vi "Main_FPGA 4.vi"() -> ()   [LabVIEW 2015]
uses:
  <vilib>/LabVIEW Targets/FPGA/cRIO/shared/nicrio_ModuleControls/nicrio_cRIO-9232_ConfigModeRing.ctl
  <vilib>/rvi/Emulation/niFpgaGetClockAttributes.vi
  <vilib>/rvi/Emulation/niFpgaSctlEmulationGetInTimedLoop.vi
  <vilib>/rvi/Emulation/niFpgaEmulationReportErrorSimple.vi
  <vilib>/rvi/Emulation/niFpgaProcessEmulError.vi
  <vilib>/rvi/eio/common/nirviEmuTemplateMethod_errors.vi
  <vilib>/rvi/interface/RandomDataEmulation/niFpgaRandomDataHandleErrors.vi
  <vilib>/rvi/Emulation/niFpgaCriticalErrorInLSC.vi
  <vilib>/eio/EIONode/EIONode.xnode
  <vilib>/rvi/DataTransferAndStorage/Container/XNode/niFpgaContainer.xnode
  <vilib>/rvi/interface/RandomDataEmulation/nirviRandomDataFpgaReadWriteTemplate.vi
  <vilib>/addons/InsightCM/Devices/Shared/AcquireBOP/FPGA/subVIs/VibAPI/BOP_VibAPI_6.lvlib
panel:
  out "Loop delay (us)":u32
  out "Chassis Temperature":sgl
  in  "Custom Scale Intercept":sgl[](array[numeric])=[0.0, 0.0, 0.0, 0.0, 0.0, 0.0, 0.0, 0.0, 0.0, 0.0, 0.0, 0.0, 0.0, 0.0, 0.0, 0.0, 0.0, 0.0, 0.0, 0.0, 0.0, 0.0, 0.0, 0.0, 0.0, 0.0, 0.0, 0.0, 0.0, 0.0, 0.0, 0.0, 0.0, 0.0, 0.0, 0.0, 0.0, 0.0, 0.0, 0.0, 0.0, 0.0, 0.0, 0.0, 0.0, 0.0, 0.0, 0.0, 0.0, 0.0, 0.0, 0.0, 0.0, 0.0, 0.0, 0.0, 0.0, 0.0, 0.0, 0.0, 0.0, 0.0, 0.0, 0.0, 0.0, 0.0, 0.0, 0.0, 0.0, 0.0, 0.0, 0.0, 0.0, 0.0, 0.0, 0.0, 0.0, 0.0, 0.0, 0.0, 0.0, 0.0, 0.0, 0.0, 0.0, 0.0, 0.0, 0.0, 0.0, 0.0, 0.0, 0.0, 0.0, 0.0, 0.0, 0.0, 0.0, 0.0, 0.0, 0.0, 0.0, 0.0, 0.0, 0.0, 0.0, 0.0, 0.0, 0.0, 0.0, 0.0, 0.0, 0.0, 0.0, 0.0, 0.0, 0.0, 0.0, 0.0, 0.0, 0.0, 0.0, 0.0, 0.0, 0.0, 0.0, 0.0, 0.0, 0.0]
  out "FPGA Error":errorcluster
  out "Finished":bool
  in  "Stop":bool
  out "Module Underflow":bool
  out "DMA FIFO Full":bool
  out "Chan Count":bool
  out "Acq Loop Ticks":u32
  out "First Read":bool
  in  "Total Avail Channels":i32=4
  in  "Data Rate [S/s]":u32=1280
  in  "Custom Scale Slope":sgl[](array[numeric])=[0.0, 0.0, 0.0, 0.0, 0.0, 0.0, 0.0, 0.0, 0.0, 0.0, 0.0, 0.0, 0.0, 0.0, 0.0, 0.0, 0.0, 0.0, 0.0, 0.0, 0.0, 0.0, 0.0, 0.0, 0.0, 0.0, 0.0, 0.0, 0.0, 0.0, 0.0, 0.0, 0.0, 0.0, 0.0, 0.0, 0.0, 0.0, 0.0, 0.0, 0.0, 0.0, 0.0, 0.0, 0.0, 0.0, 0.0, 0.0, 0.0, 0.0, 0.0, 0.0, 0.0, 0.0, 0.0, 0.0, 0.0, 0.0, 0.0, 0.0, 0.0, 0.0, 0.0, 0.0, 0.0, 0.0, 0.0, 0.0, 0.0, 0.0, 0.0, 0.0, 0.0, 0.0, 0.0, 0.0, 0.0, 0.0, 0.0, 0.0, 0.0, 0.0, 0.0, 0.0, 0.0, 0.0, 0.0, 0.0, 0.0, 0.0, 0.0, 0.0, 0.0, 0.0, 0.0, 0.0, 0.0, 0.0, 0.0, 0.0, 0.0, 0.0, 0.0, 0.0, 0.0, 0.0, 0.0, 0.0, 0.0, 0.0, 0.0, 0.0, 0.0, 0.0, 0.0, 0.0, 0.0, 0.0, 0.0, 0.0, 0.0, 0.0, 0.0, 0.0, 0.0, 0.0, 0.0, 0.0]
  in  "Acquisition Type":enum16{"Finite Samples", "Continuous Samples"}(ring)
  in  "Samps per Chan [Finite]":i32=5120
  in  "Input Config Array":T1[](array[typedef])=[0, 0, 0, 0, 0, 0, 0, 0, 0, 0, 0, 0, 0, 0, 0, 0, 0, 0, 0, 0, 0, 1, 1, 1] items=["AC Coupled", "DC Coupled", "IEPE AC Coupled"]
  in  "Number of Modules":i16=1
  in  "Enable Chan Array":bool[](array[boolean])
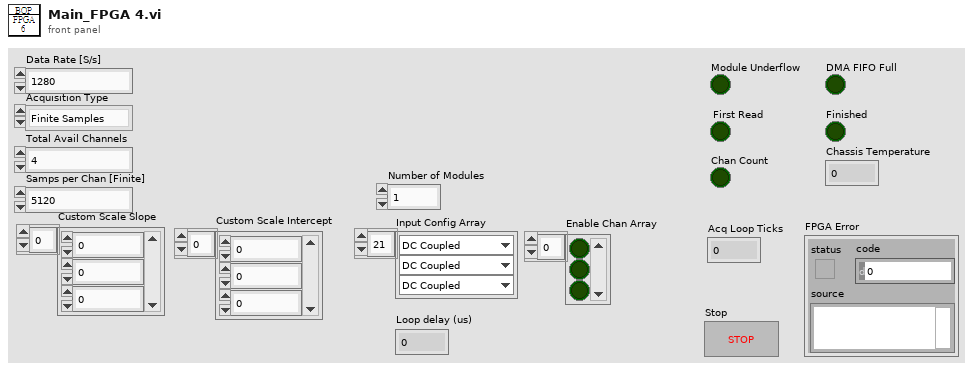
[diagram p1: front panel]
types:
  T1 = typedef "nicrio_cRIO-9232_ConfigModeRing.ctl" = u8
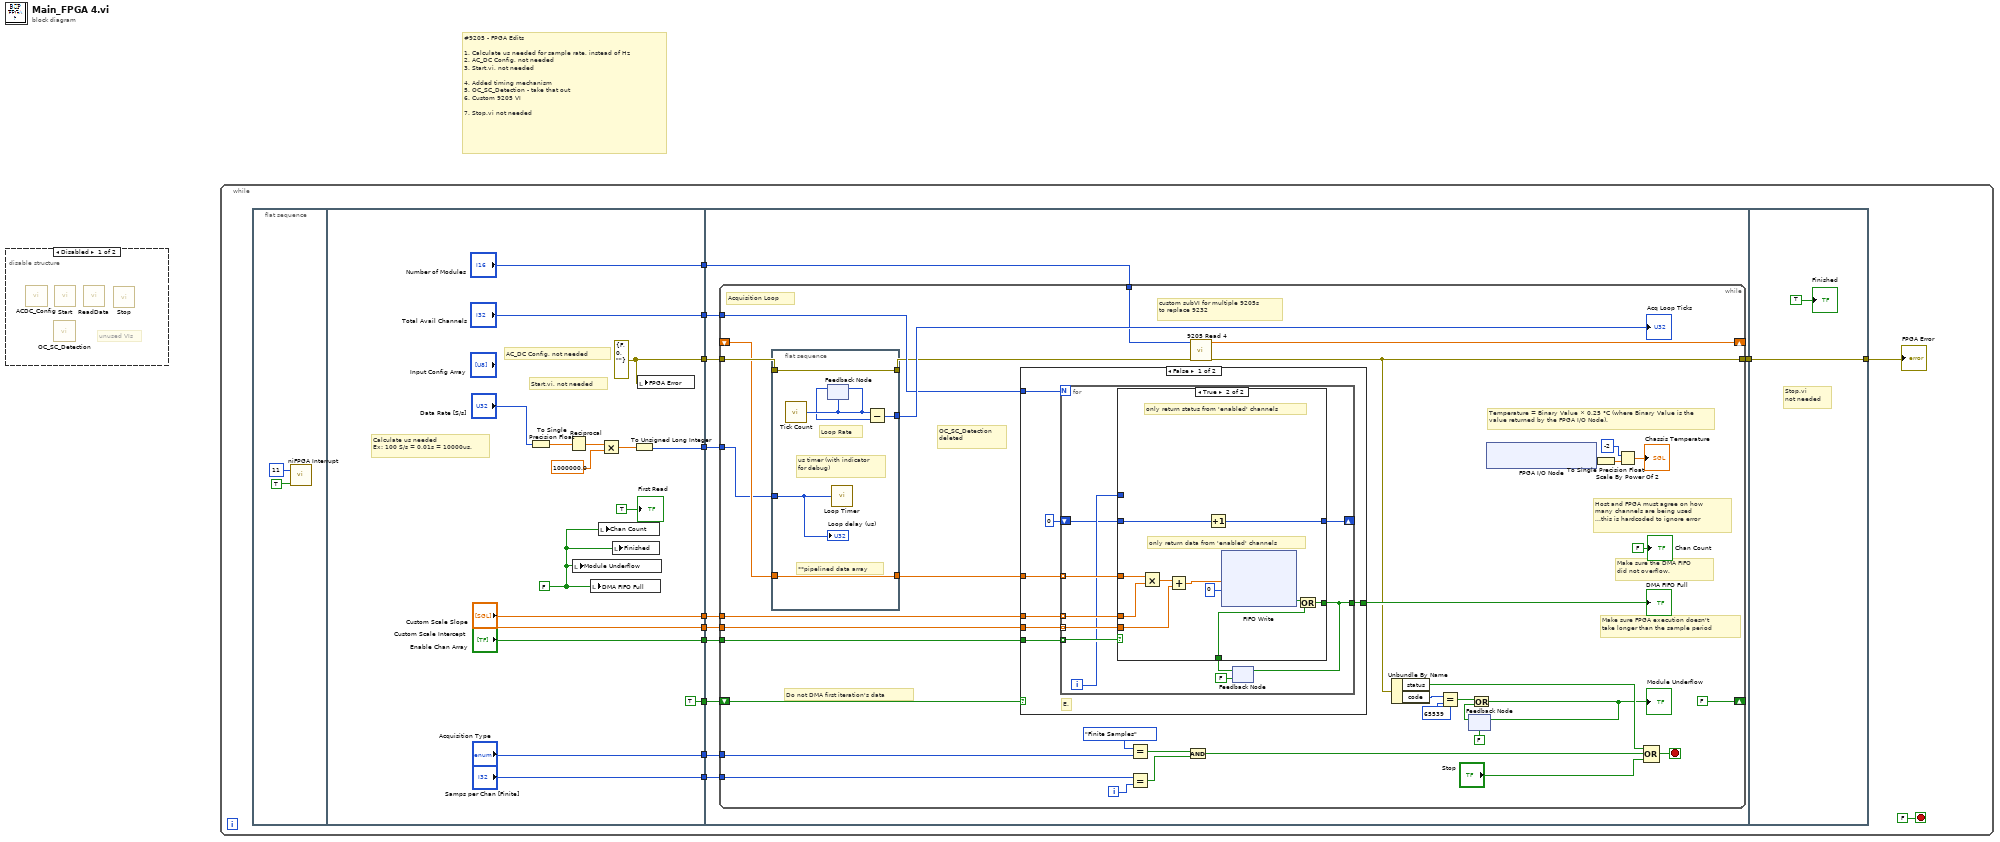
[diagram p0: block diagram]
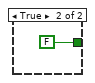
[diagram p4: hidden frame]
diagram:
  # "#9205 - FPGA Edits\n\n1. Calculate us needed for sample rate, instead of Hz\n2. AC_DC Config, not needed\n3. Start.vi, not needed\n\n4. Added timing mechanism\n5. OC_SC_Detection - take that out\n6. Custom 9205 VI\n\n7. Stop.vi not needed"
  n1 = disable-structure shown="Disabled" {
    frame Disabled {
      # "unused VIs"
      n2 = call <vilib>:"ACDC_Config.vi"() -> ()  [unwired: 11 in, 1 out]
      n3 = call <vilib>:"OC_SC_Detection.vi"() -> ()  [unwired: 10 in, 2 out]
      n4 = call <vilib>:"Start.vi"() -> ()  [unwired: 11 in, 1 out]
      n5 = call <vilib>:"ReadData.vi"() -> ()  [unwired: 10 in, 2 out]
      n6 = call <vilib>:"Stop.vi"() -> ()  [unwired: 11 in, 1 out]
    }
    frame Enabled {
    }
  }
  n7 = while {
    stop <- FALSE stop-if-true
    n8 = flat-sequence {
      tunnel: [w22] -> w12
      tunnel: ["Custom Scale Slope"] -> w11
      tunnel: ["Acquisition Type"] -> w10
      tunnel: ["Samps per Chan [Finite]"] -> w9
      tunnel: ["Total Avail Channels"] -> w8
      tunnel: [TRUE ("t")] -> w7
      tunnel: ["Number of Modules"] -> w5
      tunnel: ["Enable Chan Array"] -> w4
      tunnel: ["Custom Scale Intercept"] -> w2
      tunnel: [w16] -> w1
      tunnel: w12 -> [w42]
      tunnel: w11 -> [w41]
      tunnel: w10 -> [w39]
      tunnel: w9 -> [w38]
      tunnel: w8 -> [w43]
      tunnel: w7 -> [w40]
      tunnel: [w37] -> w6
      tunnel: w5 -> [w36]
      tunnel: w4 -> [w35]
      tunnel: w2 -> [w34]
      tunnel: w1 -> [w33]
      tunnel: w6 -> [w118]
      tunnel: [w118] -> w3
      frame #0 {
        n9 = call <vilib>:"niFPGA Interrupt.vi"("Wait Until Cleared (F)"=TRUE ("Wait Until Cleared"), "IRQ Number (0)"=u8 11 ("IRQ Number")) -> ()  [unwired: 1 in]
      }
      frame #1 {
        w22 = errorcluster {"status"=FALSE, "code"=0, "source"=""} ("FPGA Error")
        w27 = FALSE ("Module Underflow")
        # "Start.vi, not needed"
        # "AC_DC Config, not needed"
        # "Calculate us needed\nEx: 100 S/s = 0.01s = 10000us."
        n10 = To Single Precision Float(number="Data Rate [S/s]") -> (single precision float=w19:sgl)
        n11 = Reciprocal(x=w19) -> (1/x=w21:sgl)
        n12 = local write "Module Underflow"(w27) -> ()
        n13 = local write "DMA FIFO Full"(w27) -> ()
        n14 = local write "Chan Count"(w27) -> ()
        n15 = Multiply(x=w21, y=sgl 1000000.0) -> (x*y=w17:sgl)
        n16 = local write "Finished"(w27) -> ()
        n17 = To Unsigned Long Integer(number=w17) -> (unsigned 32bit integer=w16:u32)
        n18 = local write "FPGA Error"(w22) -> ()
        "First Read" <- TRUE ("First Read")
      }
      frame #2 {
        n19 = while {
          tunnel: w42 -> [w74]
          tunnel: [w46] -> w37
          tunnel: w39 -> [w76]
          tunnel: w38 -> [w75]
          shift-right: [w44] -> _
          shift-left: _ -> [w72]
          tunnel: w43 -> [w56]
          tunnel: w41 -> [w55]
          shift-right: [FALSE ("t")] -> _
          shift-left: w40 -> [w59]
          tunnel: w36 -> [w45]
          tunnel: w35 -> [w54]
          tunnel: w34 -> [w53]
          tunnel: w33 -> [w48]
          i -> [w70]
          stop <- w79 stop-if-true
          # "custom subVI for multiple 9205s\nto replace 9232"
          # "OC_SC_Detection\ndeleted"
          # "Temperature = Binary Value × 0.25 °C (where Binary Value is the value returned by the FPGA I/O Node)."
          # "Do not DMA first iteration's data"
          # "Acquisition Loop"
          # "Host and FPGA must agree on how \nmany channels are being used\n...this is hardcoded to ignore error"
          # "Make sure the DMA FIFO\ndid not overflow."
          # "Make sure FPGA execution doesn't\ntake longer than the sample period"
          n20 = flat-sequence {
            tunnel: [w117] -> w47
            tunnel: w74 -> [w117]
            tunnel: [w114] -> w73
            tunnel: w72 -> [w113]
            tunnel: [w113] -> w57
            tunnel: w48 -> [w112]
            frame #0 {
              # "us timer (with indicator\nfor debug)"
              # "**pipelined data array"
              # "Loop Rate"
              n21 = call "Tick Count"() -> ("Tick Count(Ticks)"=w116:u32)
              n22 = feedback-in #1(w116) -> ()
              n23 = feedback #1(w116) -> (w115:u32)
              n24 = call "Loop Timer"("Count(uSec)"=w112) -> ()  [unwired: 1 out]
              n25 = Subtract(x=w116, y=w115) -> (x-y=w114:u32)
              "Loop delay (us)" <- w112
            }
          }
          n26 = case shown="False" w59 {
            tunnel: [w87 FALSE] -> w58
            tunnel: w55 -> [w86 _]
            tunnel: w57 -> [w85 _]
            tunnel: w56 -> [w84 _]
            tunnel: w54 -> [w83 _]
            tunnel: w53 -> [w82 _]
            frame False {
              # "E."
              n27 = for {
                N: w84 -> [_]
                tunnel: [w96] -> w87
                tunnel: w85 -> [w95] mode=indexing
                tunnel: w86 -> [w94] mode=indexing
                tunnel: w83 -> [w92] mode=indexing
                tunnel: w82 -> [w91] mode=indexing
                shift-right: [w88] -> _
                shift-left: 0 -> [w89]
                i -> [w90]
                n28 = feedback #2(FALSE) -> (w97:bool)
                n29 = case shown="True" w92 {
                  tunnel: w97 -> [w99 w110]
                  tunnel: [w99 w109] -> w96
                  tunnel: w95 -> [_ w108]
                  tunnel: w94 -> [_ w107]
                  tunnel: w91 -> [_ w102]
                  tunnel: w90 -> [_ _]
                  tunnel: w89 -> [w98 w101]
                  tunnel: [w98 w100] -> w88
                  frame False {
                  }
                  frame True {
                    # "only return status from 'enabled' channels"
                    # "only return data from 'enabled' channels"
                    n30 = Multiply(x=w108, y=w107) -> (x*y=w104:sgl)
                    n31 = Add(x=w104, y=w102) -> (x+y=w103:sgl)
                    n32 = Increment(x=w101) -> (x+1=w100:i32)
                    n33 = xnode ("FIFO Write")("Element"=w103, "Timeout"=0) -> ("Timed Out?"=w105:bool)  [unwired: 1 in, 1 out]
                    n34 = Or(x=w105, y=w110) -> (x .or. y?=w109:bool)
                  }
                }
                n35 = feedback-in #2(w96) -> ()
              }
            }
            frame True {
            }
          }
          "DMA FIFO Full" <- w58
          n36 = Equal?(x=enum16{"Finite Samples", "Continuous Samples"}."Finite Samples" ("y"), y=w76) -> (x = y?=w64:bool)
          n37 = Equal?(x=w75, y=w70) -> (x = y?=w63:bool)
          n38 = And(x=w64, y=w63) -> (x .and. y?=w62:bool)
          n39 = call "9205 Read 4.vi"("error in"=w47, "Module Config Selector"=w45) -> ("error out"=w46:errorcluster, "Data Array"=w44:sgl[])  [unwired: 8 in]
          n40 = Unbundle By Name(w46) -> ("status"=w69:bool, "code"=w77:i32)
          n41 = Equal?(x=w77, y=65539) -> (x = y?=w66:bool)
          n42 = feedback #3(FALSE) -> (w68:bool)
          n43 = Or(x=w66, y=w68) -> (x .or. y?=w65:bool)
          "Module Underflow" <- w65
          n44 = feedback-in #3(w65) -> ()
          n45 = xnode "FPGA I/O Node"() -> ("Chassis Temperature"=w50:i16)  [unwired: 1 in, 1 out]
          n46 = To Single Precision Float(number=w50) -> (single precision float=w52:sgl)
          n47 = Scale By Power Of 2(n=i16 -2, x=w52) -> (x*2^n=→"Chassis Temperature":sgl)
          n48 = Compound Arithmetic op=OR(w69, w62, "Stop") -> (w79:bool)
          "Chan Count" <- FALSE ("Chan Count")
          "Acq Loop Ticks" <- w73
        }
      }
      frame #3 {
        # "Stop.vi\nnot needed"
        "Finished" <- TRUE ("Finished")
      }
    }
    "FPGA Error" <- w3
  }
